vi "Set Splitter Size (Core).vi"(8 "error in (no error)":errorcluster, 10 "Size":i32, 11 "Splitter in":refnum<class "Splitter.lvclass">) -> (0 "error out":errorcluster, 3 "Splitter out":refnum<class "Splitter.lvclass">)   [LabVIEW 2017, in "Splitter.lvclass"]
uses:
  Splitter.lvclass
  Splitter.lvclass/Splitter.ctl
  Low-Level VI Manipulation/Find Resource by Type (String).vi
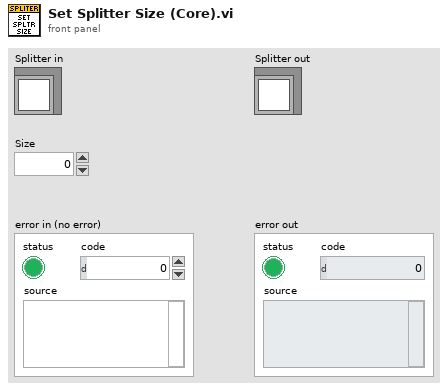
[diagram p1: front panel]
types:
  T1 = typedef "Resource Array.ctl" = T2[]
  T2 = typedef "Resource.ctl" = cluster{"type":u32, "id":i32, "name":string, "binary data":string}
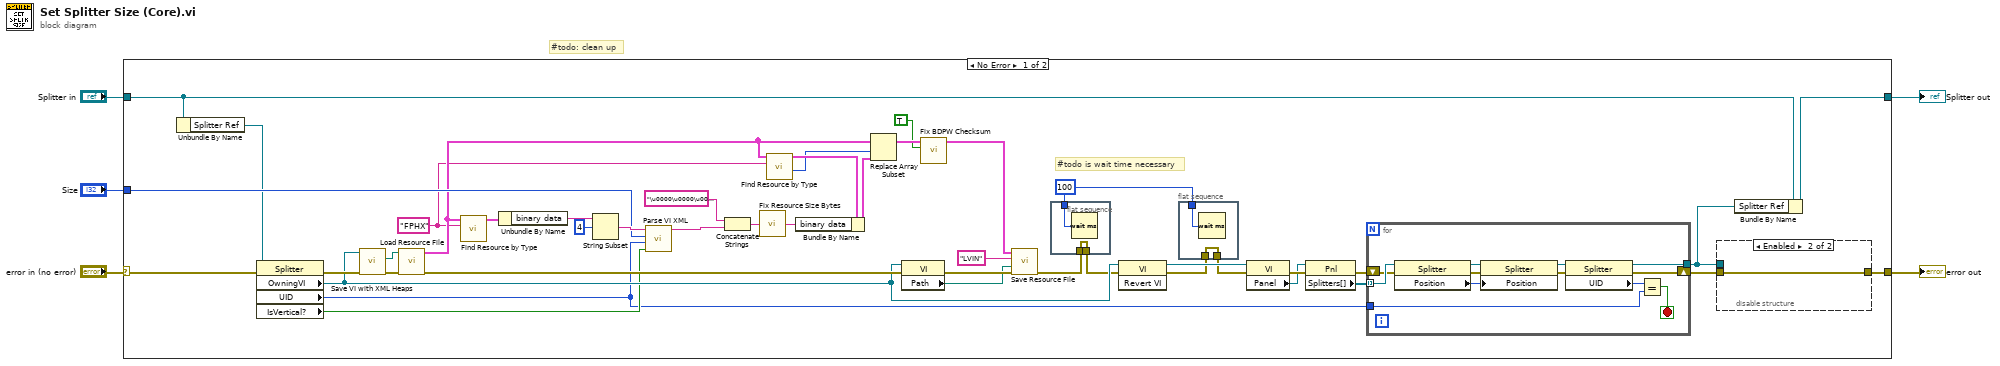
[diagram p0: block diagram]
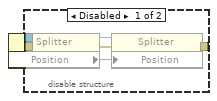
[diagram p2: hidden frame]
diagram:
  # "#todo: clean up"
  n1 = case shown="No Error" "error in (no error)" {
    selector: "error in (no error)" -> [w44 w73]
    tunnel: [w23 w73] -> w4
    tunnel: [w13 w74] -> w2
    tunnel: "Splitter in" -> [w12 w74]
    tunnel: "Size" -> [w41 _]
    frame No Error {
      w10 = u32 100 ("milliseconds to wait")
      w24 = "FPHX"
      # "#todo is wait time necessary"
      n2 = Unbundle By Name(w12) -> ("Splitter Ref"=w14:refnum<vi>)
      n3 = property class="Splitter"(reference=w14, error in=w44) -> (error out=w42:errorcluster, "OwningVI"=w25:refnum<vi>, "UID"=w16:i32, "IsVertical?"=w17:bool)  [unwired: 1 out]
      n4 = call "Save VI with XML Heaps.vi"("error in (no error)"=w42, "VI Refnum In"=w25) -> ("error out"=w45:errorcluster, "VI Path out"=w49:path)  [unwired: 7 in, 1 out]
      n5 = call "Load Resource File.vi"("error in (no error)"=w45, "Resource file"=w49) -> ("error out"=w31:errorcluster, "Resources"=w29:T1)  [unwired: 7 in, 1 out]
      n6 = call-poly "Find Resource by Type.vi"("Resource Type"=w24, "Resources"=w29) -> ("Resource"=w46:T2)  [unwired: 7 in, 2 out]
      n7 = Unbundle By Name(w46) -> ("binary data"=w47:string)
      n8 = String Subset(string=w47, offset (0)=4) -> (substring=w43:string)  [unwired: 1 in]
      n9 = call "Parse VI XML.vi"("Is Vertical?"=w17, "UID"=w16, "New Size"=w41, "VI XML"=w43) -> ("VI XML With New Size"=w30:string)  [unwired: 6 in, 1 out]
      n10 = Concatenate Strings("\u0000\u0000\u0000\u0000", w30) -> (w39:string)
      n11 = call "Fix Resource Size Bytes.vi"("Data In"=w39) -> ("Data Out"=w38:string)
      n12 = call-poly "Find Resource by Type.vi"("Resource Type"=w24, "Resources"=w29) -> ("Index"=w36:i32, "Resource"=w37:T2)  [unwired: 7 in, 1 out]
      n13 = Bundle By Name(cluster=w37, "binary data"=w38) -> (w35:T2)
      n14 = Replace Array Subset(array=w29, new element=w35, index=w36) -> (w34:T1)
      n15 = property class="VI"(reference=w25, error in=w31) -> (error out=w27:errorcluster, "Path"=w26:path)  [unwired: 1 out]
      n16 = call "Fix BDPW Checksum.vi"("Only fix 3rd hash (F)"=TRUE, "Resources in"=w34) -> ("Resources out"=w33:T1)  [unwired: 9 in]
      n17 = call "Save Resource File.vi"("error in (no error)"=w27, "Path"=w26, "File type"="LVIN", "Resources"=w33) -> ("error out"=w8:errorcluster)  [unwired: 7 in]
      n18 = flat-sequence {
        tunnel: w10 -> [w53]
        tunnel: [w52] -> w9
        tunnel: w8 -> [w52]
        frame #0 {
          n19 = Wait (ms)(milliseconds to wait=w53) -> ()  [unwired: 1 out]
        }
      }
      n20 = invoke class="VI" method="Revert VI"(reference=w25, error in=w9) -> (reference out=w22:refnum<vi>, error out=w6:errorcluster)  [unwired: 1 in, 1 out]
      n21 = flat-sequence {
        tunnel: w10 -> [w51]
        tunnel: [w50] -> w7
        tunnel: w6 -> [w50]
        frame #0 {
          n22 = Wait (ms)(milliseconds to wait=w51) -> ()  [unwired: 1 out]
        }
      }
      n23 = property class="VI"(reference=w22, error in=w7) -> (error out=w21:errorcluster, "Panel"=w20:refnum<vi>)  [unwired: 1 out]
      n24 = property class="Pnl"(reference=w20, error in=w21) -> (error out=w19:errorcluster, "Splitters[]"=w18:refnum<vi>[])  [unwired: 1 out]
      n25 = for {
        tunnel: w18 -> [w63] mode=indexing
        tunnel: w16 -> [w71]
        shift-right: [w69] -> w15
        shift-left: w19 -> [w61]
        tunnel: [w68] -> w11
        stop <- w70 stop-if-true
        n26 = property class="Splitter"(reference=w63, error in=w61) -> (reference out=w66:refnum<vi>, error out=w67:errorcluster, "Position"=w65:i32)
        n27 = property class="Splitter"(reference=w66, error in=w67, "Position"=w65) -> (reference out=w64:refnum<vi>, error out=w62:errorcluster)
        n28 = property class="Splitter"(reference=w64, error in=w62) -> (reference out=w68:refnum<vi>, error out=w69:errorcluster, "UID"=w72:i32)
        n29 = Equal?(x=w72, y=w71) -> (x = y?=w70:bool)
      }
      n30 = disable-structure shown="Enabled" {
        disable-tunnel: [w56 w60] -> w23
        disable-tunnel: w15 -> [w55 w60]
        disable-tunnel: w11 -> [w54 _]
        frame Disabled {
          n31 = property class="Splitter"(reference=w54, error in=w55) -> (reference out=w58:refnum<vi>, error out=w57:errorcluster, "Position"=w59:i32)
          n32 = property class="Splitter"(reference=w58, error in=w57, "Position"=w59) -> (error out=w56:errorcluster)  [unwired: 1 out]
        }
        frame Enabled {
        }
      }
      n33 = Bundle By Name(cluster=w12, "Splitter Ref"=w11) -> (w13:refnum<class "Splitter.lvclass">)
    }
    frame Error {
    }
  }
  "error out" <- w4
  "Splitter out" <- w2
